vi "Create File if Do Not Exist.vi"(8 "ErrorIn":errorcluster, 9 "FileName":string, 10 "FolderName":string, 11 "LogsClass In":refnum<class "Logs.lvclass">) -> (0 "ErrorOut":errorcluster, 3 "LogClass Out":refnum<class "Logs.lvclass">)   [LabVIEW 2019, in "Logs.lvclass"]
uses:
  Logs.lvclass
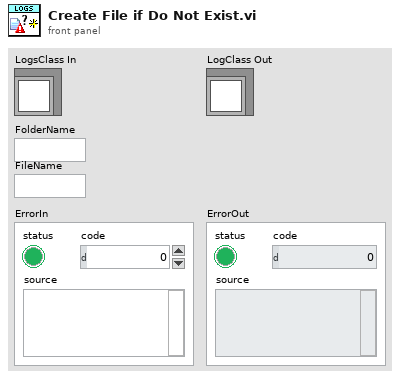
[diagram p1: front panel]
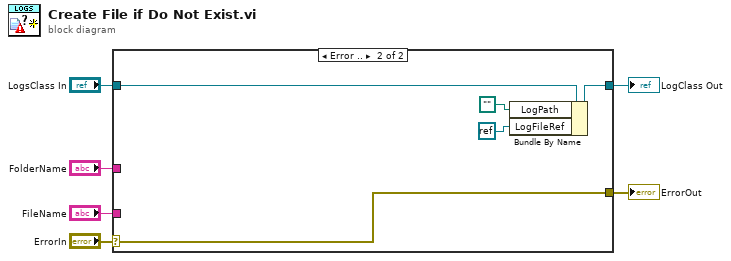
[diagram p0: block diagram]
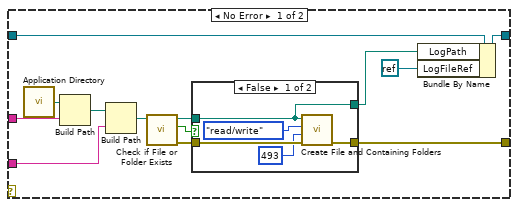
[diagram p2: hidden frame]
diagram:
  n1 = case shown="Error .." "ErrorIn" {
    selector: "ErrorIn" -> [_ w31]
    tunnel: "FolderName" -> [w18 _]
    tunnel: "FileName" -> [w17 _]
    tunnel: [w11 w31] -> w4
    tunnel: [w9 w29] -> w2
    tunnel: "LogsClass In" -> [w10 w30]
    frame No Error {
      n2 = call <vilib>:"Application Directory.vi"() -> ("Application Directory"=w19:path)
      n3 = Build Path(base path=w19, name or relative path=w18) -> (appended path=w16:path)
      n4 = Build Path(base path=w16, name or relative path=w17) -> (appended path=w12:path)
      n5 = call <vilib>:"Check if File or Folder Exists.vi"("path"=w12) -> ("error out"=w15:errorcluster, "file or folder exists?"=w13:bool, "dup path"=w14:path)  [unwired: 8 in]
      n6 = case shown="False" w13 {
        tunnel: w14 -> [w22 w25]
        tunnel: w15 -> [w24 w26]
        tunnel: [w23 w26] -> w11
        tunnel: [w22 w25] -> w8
        frame False {
          n7 = call <vilib>:"Create File and Containing Folders.vi"("error in (no error)"=w24, "permissions"=i16 493, "access"=enum16{"read/write", "read-only", "write-only"}."read/write", "file path"=w22) -> ("error out"=w23:errorcluster)  [unwired: 6 in, 1 out]
        }
        frame True {
        }
      }
      n8 = Bundle By Name(cluster=w10, "LogPath"=w8, "LogFileRef"=refnum<k0> refnum) -> (w9:refnum<class "Logs.lvclass">)
    }
    frame Error {
      n9 = Bundle By Name(cluster=w30, "LogPath"=path "", "LogFileRef"=refnum<k0> refnum) -> (w29:refnum<class "Logs.lvclass">)
    }
  }
  "ErrorOut" <- w4
  "LogClass Out" <- w2
